vi "5.4.1.vi"(9 "난이도":dbl, 10 "독창성":dbl, 11 "창의력":dbl) -> (3 "숫자형":dbl)   [LabVIEW 2018]
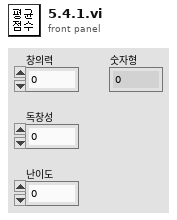
[diagram p1: front panel]
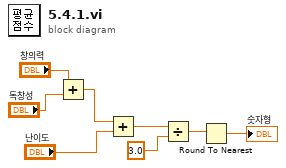
[diagram p0: block diagram]
diagram:
  n1 = Add(x="창의력", y="독창성") -> (x+y=w3:dbl)
  n2 = Add(x=w3, y="난이도") -> (x+y=w5:dbl)
  n3 = Divide(x=w5, y=3.0 ("x")) -> (x/y=w6:dbl)
  n4 = Round To Nearest(number=w6) -> (nearest integer value=→"숫자형":dbl)
